vi "[ToBeTest] Complete Measurament RT.vi"() -> ()   [LabVIEW 2014]
uses:
  <vilib>/Platform/TimedLoop/XDataNode/timing_clust.ctl
  <vilib>/Platform/TimedLoop/XDataNode/nitl_modes.ctl
  <vilib>/Platform/TimedLoop/XDataNode/wakeup.ctl
  <vilib>/FPGAPlugInAG/sbRIO-9636/niLvFpga_Open_sbRIO-9636.vi
  <vilib>/rvi/interface/common/dynamic/niFpgaDynamicAddResources.vi
  <vilib>/FPGAPlugInAG/Dynamic/niLvFpga_Reset_Dynamic.vi
  <vilib>/Utility/error.llb/Error Cluster From Error Code.vi
  <vilib>/rvi/errors/niLvFpgaAdjustHostInterfaceError.vi
  <vilib>/rvi/interface/common/niFpgaWaitOnOcc.vi
  <vilib>/FPGAPlugInAG/Dynamic/niLvFpga_Run_Dynamic.vi
  <vilib>/FPGAPlugInAG/Dynamic/niLvFpga_Abort_Dynamic.vi
  <vilib>/FPGAPlugInAG/Dynamic/niLvFpga_Close_Dynamic.vi
  <vilib>/rvi/interface/nirviOpenFPGA/nirviOpenFPGA.xnode
  FPGA Bitfiles/LaserDistanceSen_FPGATarget_N-ParametricDoub_YVLbjAYtdP4.lvbitx
  FPGA Target/Test VIs/N-Parametric Double FFT Mesurament Test.vi
  <vilib>/rvi/interface/nirviMethod/nirviMethod.xnode
  <vilib>/rvi/interface/nirviReadWriteControl/nirviReadWriteControl.xnode
  <vilib>/platform/TimedLoop/XDataNode/XDataNode.xnode
  <vilib>/rvi/interface/nirviCloseFPGA/nirviCloseFPGA.xnode
  <vilib>/FPGAPlugInAG/Dynamic/niLvFpga_ConfigureFifo_Dynamic.vi
  <vilib>/rvi/errors/niLvFpgaMergeErrorWithErrorCode.vi
  <vilib>/FPGAPlugInAG/Dynamic/niLvFpga_StartFifo_Dynamic.vi
  <vilib>/rvi/interface/Simulation/niFpgaSimulationCallBeginRW.vi
  <vilib>/FPGAPlugInAG/Dynamic/niLvFpga_ReadFifo_Dynamic.vi
  <vilib>/Platform/TimedLoop/XDataNode/XDNodeRunTimeDep.lvlib
  NiFpgaLv.dll
  <vilib>/Analysis/NI_AALBase.lvlib
panel:
  in  "#movesignal":i32=10
  out "moving standard deviation rel":dbl format="%0.5f"
  out "moving mean":dbl format="%0.7f"
  out "StdDev Rel 1":dbl
  out "StdDev Rel 2":dbl
  out "Warning":bool
  out "Velocity (m/s)":dbl
  out "Distance (m)":dbl
  out "Mean Frequency":dbl
  out "Rise array size":i32
  out "Fall array size":i32
  out "Mean Frequency Rising (Hz)":dbl
  out "Mean Frequency Falling (Hz)":dbl
  in  "tieni premuto per":i32=1
  in  "Triangular Multiply Factor":dbl[](array[numeric])=[1.0, 0.8, 0.95, 0.85, 0.9]
  out "RISING Second Edge N-FFT":dbl[](graph)
  in  "Enable triangular scaling":bool=TRUE
  in  "Triangolo dritto?":bool
  out "FALLING First Edge N-FFT":dbl[](graph)
  in  "#Signals":u32(slide)=5 scale=1.0..5.0
  in  "stop":bool
  in  "Initial Latency points":u32(slide) scale=0.0..1249.0
  out "Elements Remaining FFT":u32
  out "Elements Remaining Signal":u32
  out "N-Signals":dbl[](graph)
  in  "Snapshot":bool
  in  "Windowing":T1(ring)
  in  "first bin":i32=5
  in  "last bin":i32=255
  in  "lower limit 2":u32(slide)=738 scale=625.0..738.0
  in  "lower limit 1":u32(slide)=113 scale=0.0..113.0
  # "OFFLINE parameters"
  # "Max Detection FFT bin range"
  # "WARNING:\nOnce pressed wait untill the end of operation"
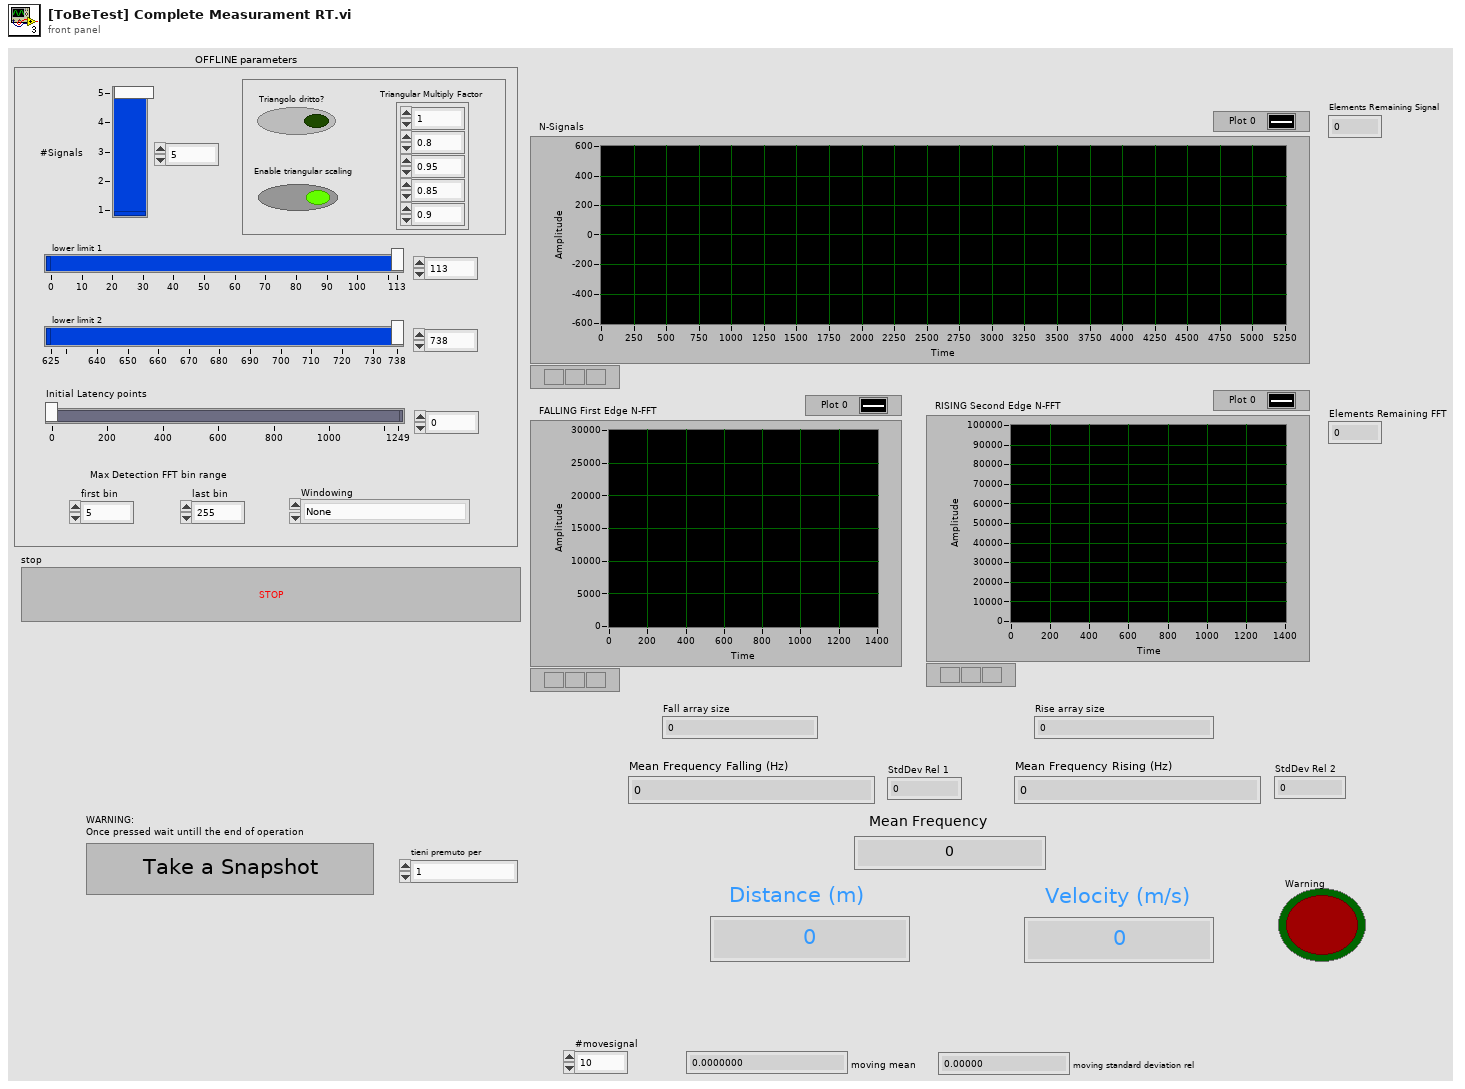
[diagram p1: front panel]
types:
  T1 = enum16{"None", "Hanning", "Hamming", "Blackman", "Blackman-Harris"}
  T2 = typedef "XDNodeRunTimeDep.lvlib/timing_clust.ctl" = cluster{"Expected End [f-1]":u64, "Actual End [f-1]":u64, "Finished Late? [f-1]":bool, "Expected End [i-1]":u64, "Actual End [i-1]":u64, "Finished Late? [i-1]":bool, "Expected Start [i]":u64, "Actual Start [i]":u64, "Expected Start [f]":u64, "Actual Start [f]":u64, "Source Name":string, "Structure Name":string, "Period":i64, "Deadline":i64, "Offset":i64, "Start":i64, "Priority":i32, "Timeout":i32, "Mode":T3, "Wakeup Reason":T4, "Error":errorcluster, "Source Type":string, "Secondary Source Type":string, "Global End Time":u64, "Global Start Time":u64, "Frame Duration":u64, "Iteration Duration":u64, "Assigned CPU":i32, "I/O Scan Engine Mode":u32}
  T3 = typedef "XDNodeRunTimeDep.lvlib/nitl_modes.ctl" = enum32{"No Change", "Process missed periods, maintain original phase", "Discard missed periods, maintain original phase", "Process missed periods, ignore original phase", "Discard missed periods, ignore original phase"}
  T4 = typedef "XDNodeRunTimeDep.lvlib/wakeup.ctl" = enum32{"Normal", "Aborted", "Asynchronous wakeup", "Timing source error", "Timed loop error", "Timeout"}
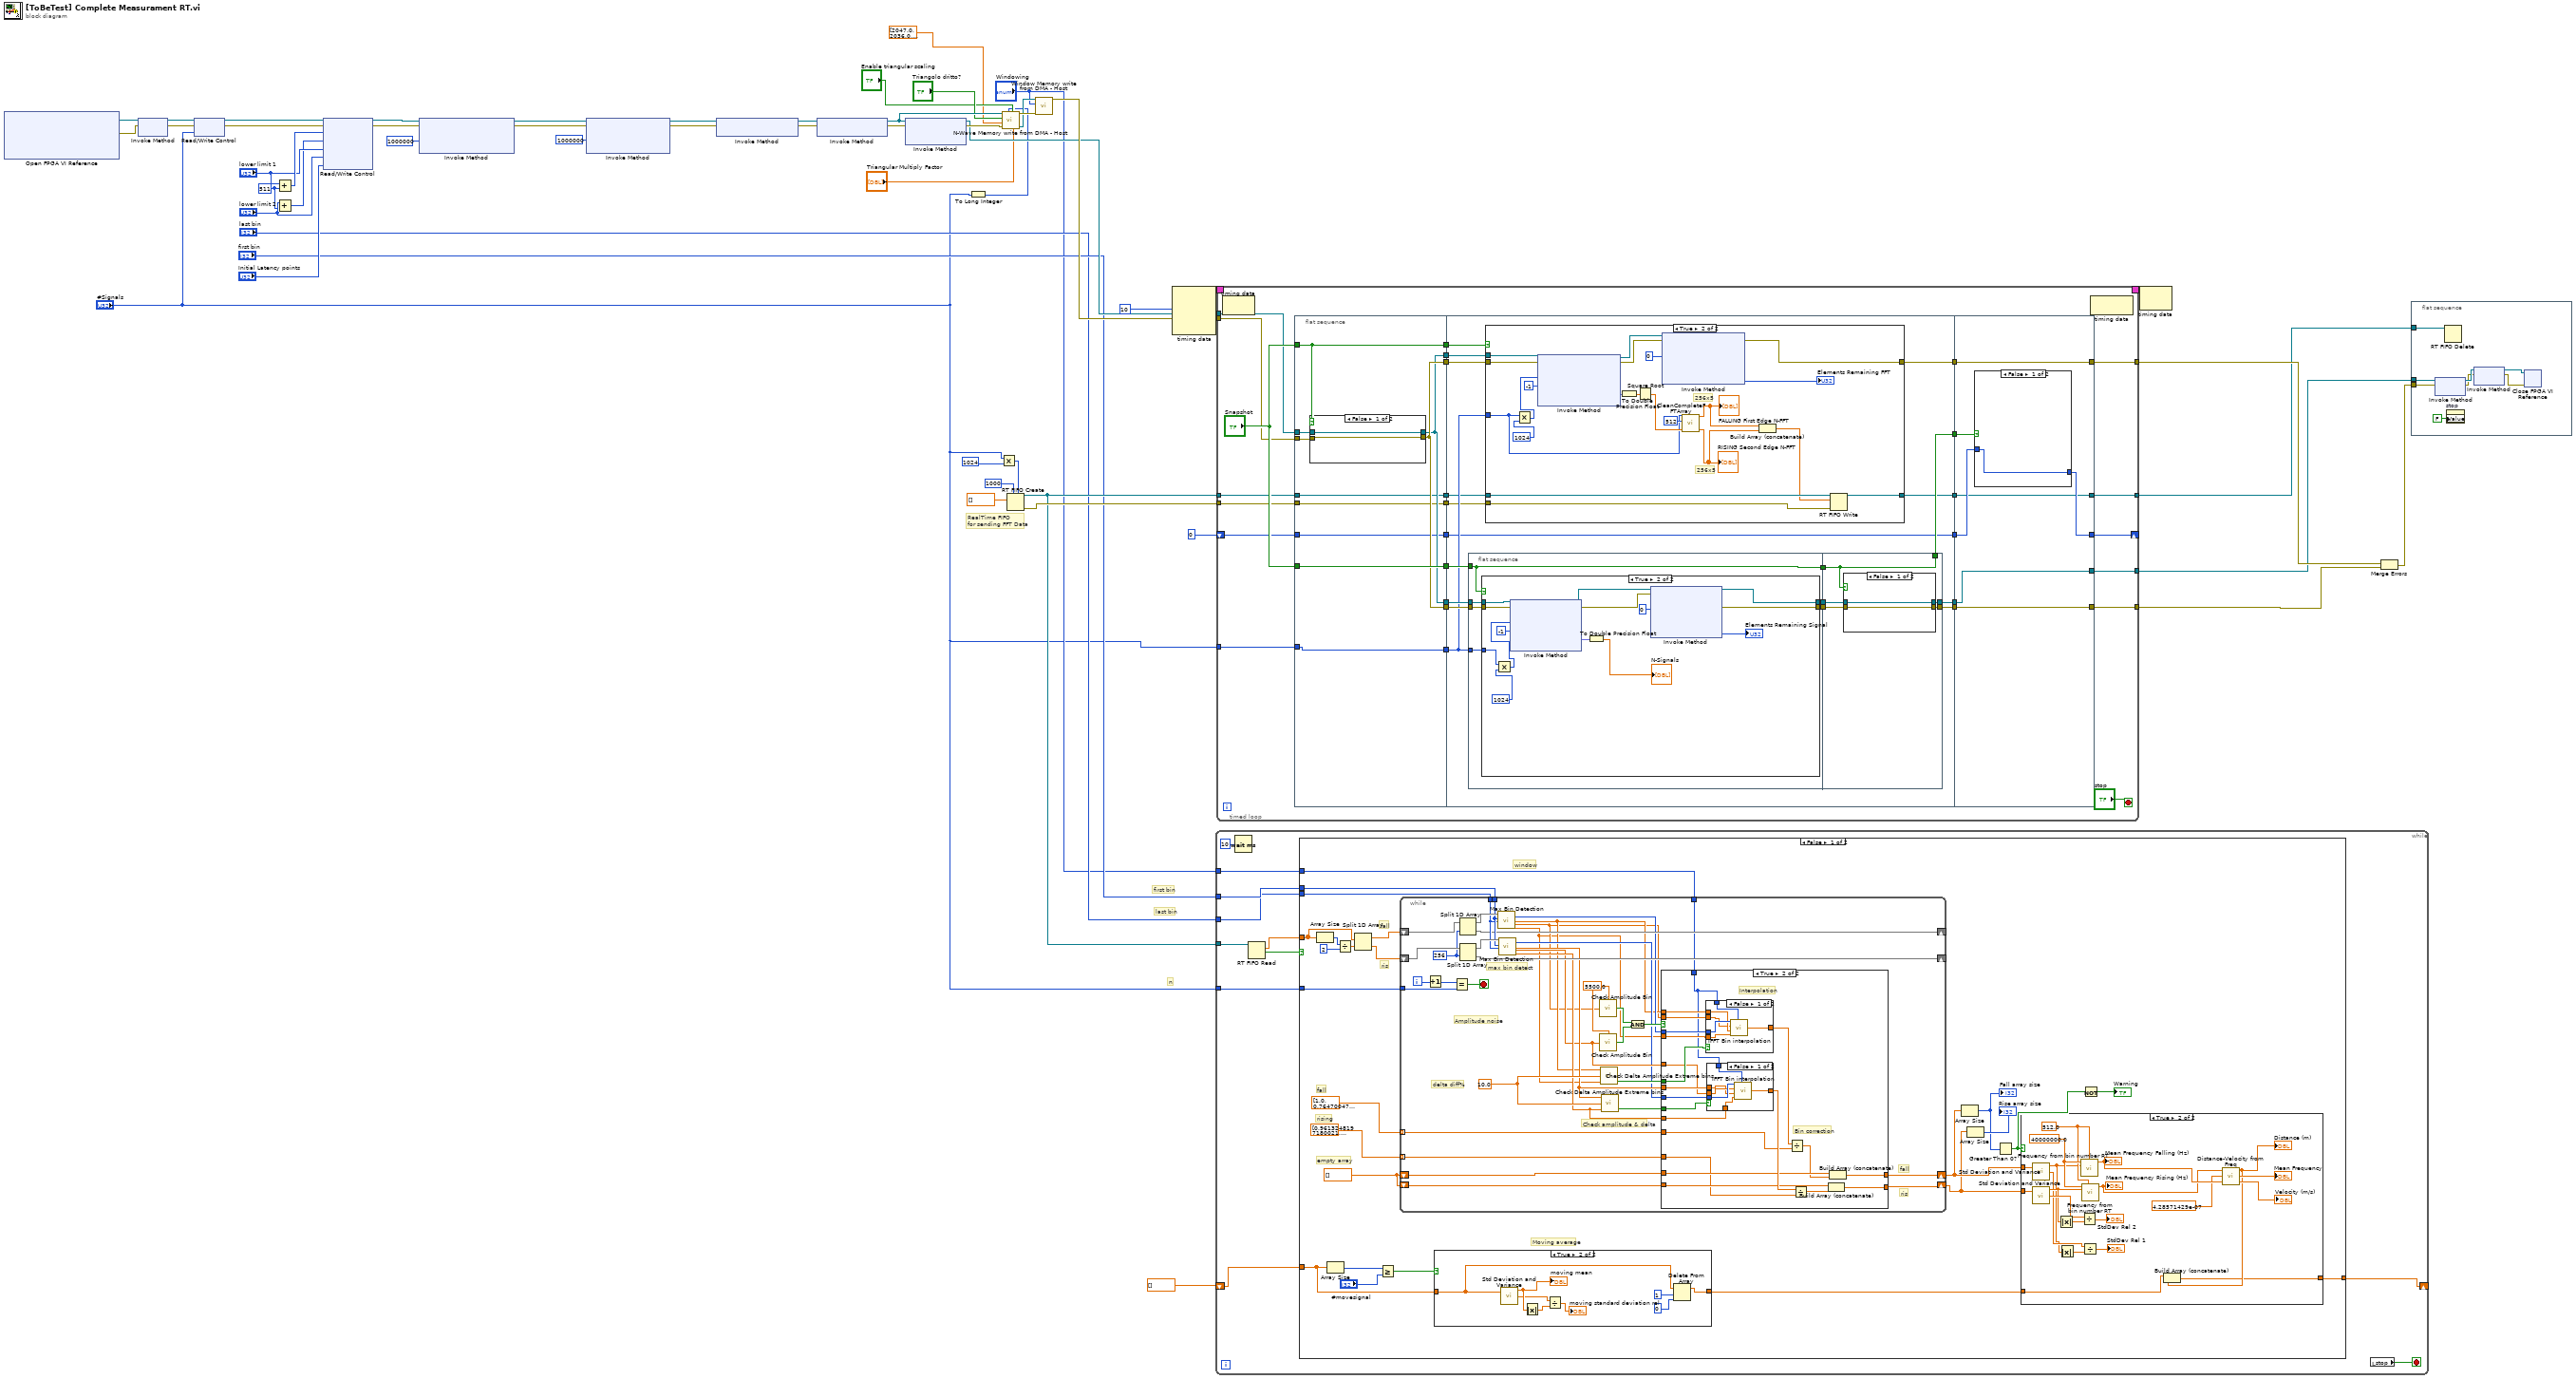
[diagram p0: block diagram]
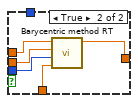
[diagram p5: hidden frame]
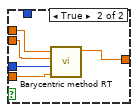
[diagram p6: hidden frame]
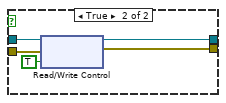
[diagram p8: hidden frame]
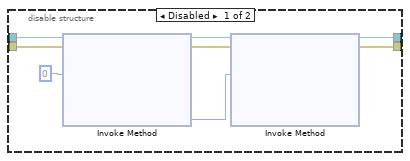
[diagram p10: hidden frame]
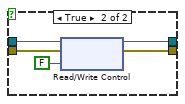
[diagram p11: hidden frame]
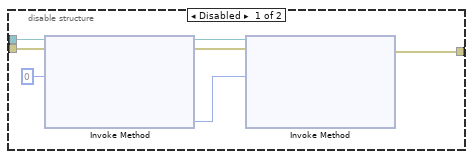
[diagram p13: hidden frame]
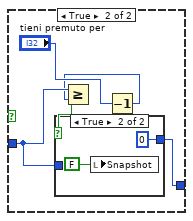
[diagram p14: hidden frame]
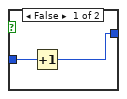
[diagram p15: hidden frame]
diagram:
  w50 = u32 511 ("y")
  # "n"
  # "last bin"
  # "first bin"
  # "RealTime FIFO \nfor sending FFT Data"
  n1 = xnode "Open FPGA VI Reference"() -> ("FPGA VI Reference Out"=w24:refnum<k20>, "error out"=w23:errorcluster)  [unwired: 2 in]
  n2 = xnode "Invoke Method"("FPGA VI Reference In"=w24, "error in"=w23) -> ("FPGA VI Reference Out"=w21:refnum<k20>, "error out"=w22:errorcluster)
  n3 = xnode "Read/Write Control"("FPGA VI Reference In"=w21, "error in"=w22, "n"="#Signals") -> ("FPGA VI Reference Out"=w20:refnum<k20>, "error out"=w19:errorcluster)
  n4 = Add(x="lower limit 1", y=w50) -> (x+y=w54:u32)
  n5 = Add(x="lower limit 2", y=w50) -> (x+y=w52:u32)
  n6 = xnode "Read/Write Control"("FPGA VI Reference In"=w20, "error in"=w19, "upper limit 1"=w54, "upper limit 2"=w52, "lower limit 1"="lower limit 1", "lower limit 2"="lower limit 2", "Latency points"="Initial Latency points") -> ("FPGA VI Reference Out"=w48:refnum<k20>, "error out"=w47:errorcluster)
  n7 = xnode "Invoke Method"("FPGA VI Reference In"=w48, "error in"=w47, "Requested Depth"=u32 1000000) -> ("FPGA VI Reference Out"=w35:refnum<k20>, "error out"=w36:errorcluster)  [unwired: 1 out]
  n8 = xnode "Invoke Method"("FPGA VI Reference In"=w35, "error in"=w36, "Requested Depth"=u32 1000000) -> ("FPGA VI Reference Out"=w42:refnum<k20>, "error out"=w43:errorcluster)  [unwired: 1 out]
  n9 = xnode "Invoke Method"("FPGA VI Reference In"=w42, "error in"=w43) -> ("FPGA VI Reference Out"=w33:refnum<k20>, "error out"=w34:errorcluster)
  n10 = xnode "Invoke Method"("FPGA VI Reference In"=w33, "error in"=w34) -> ("FPGA VI Reference Out"=w28:refnum<k20>, "error out"=w41:errorcluster)
  n11 = xnode "Invoke Method"("FPGA VI Reference In"=w28, "error in"=w41) -> ("FPGA VI Reference Out"=w29:refnum<k20>, "error out"=w32:errorcluster)  [unwired: 1 in]
  n12 = To Long Integer(number="#Signals") -> (32bit integer=w14:i32)
  n13 = Multiply(x="#Signals", y=u32 1024 ("elements in array (1)")) -> (x*y=w10:u32)
  n14 = call "N-Wave Memory write from DMA - Host.vi"("Triangular Multiply Factor"="Triangular Multiply Factor", "Enable triangular scaling"="Enable triangular scaling", "n"=w14, "error in"=w32, "Custom Triangular Signal (fal-ris)"=dbl[] [2047.0, 2036.0, 2024.0, 2013.0, 2002.0, 1990.0, 1979.0, 1968.0, 1956.0, 1945.0, 1934.0, 1923.0, 1912.0, 1900.0, 1889.0, 1878.0, 1867.0, 1856.0, 1845.0, 1833.0, 1822.0, 1811.0, 1800.0, 1789.0, 1778.0, 1767.0, 1756.0, 1745.0, 1734.0, 1723.0, 1712.0, 1702.0, 1691.0, 1680.0, 1669.0, 1658.0, 1647.0, 1636.0, 1626.0, 1615.0, 1604.0, 1593.0, 1583.0, 1572.0, 1561.0, 1550.0, 1540.0, 1529.0, 1518.0, 1508.0, 1497.0, 1487.0, 1476.0, 1465.0, 1455.0, 1444.0, 1434.0, 1423.0, 1413.0, 1402.0, 1392.0, 1381.0, 1371.0, 1360.0, 1350.0, 1340.0, 1329.0, 1319.0, 1309.0, 1298.0, 1288.0, 1278.0, 1267.0, 1257.0, 1247.0, 1237.0, 1226.0, 1216.0, 1206.0, 1196.0, 1186.0, 1176.0, 1165.0, 1155.0, 1145.0, 1135.0, 1125.0, 1115.0, 1105.0, 1095.0, 1085.0, 1075.0, 1065.0, 1055.0, 1045.0, 1035.0, 1025.0, 1015.0, 1006.0, 996.0, 986.0, 976.0, 966.0, 956.0, 947.0, 937.0, 927.0, 917.0, 908.0, 898.0, 888.0, 879.0, 869.0, 859.0, 850.0, 837.0, 826.0, 816.0, 804.0, 796.0, 788.0, 778.0, 769.0, 758.0, 750.0, 743.0, 733.0, 724.0, 717.0, 709.0, 701.0, 693.0, 686.0, 677.0, 669.0, 661.0, 653.0, 645.0, 638.0, 630.0, 622.0, 615.0, 607.0, 599.0, 592.0, 583.0, 576.0, 569.0, 561.0, 554.0, 547.0, 539.0, 532.0, 525.0, 518.0, 509.0, 501.0, 492.0, 486.0, 478.0, 471.0, 463.0, 456.0, 450.0, 442.0, 435.0, 429.0, 421.0, 415.0, 408.0, 401.0, 394.0, 388.0, 381.0, 375.0, 368.0, 361.0, 355.0, 349.0, 342.0, 336.0, 330.0, 323.0, 317.0, 311.0, 304.0, 298.0, 292.0, 286.0, 279.0, 273.0, 267.0, 261.0, 255.0, 249.0, 242.0, 236.0, 230.0, 224.0, 218.0, 212.0, 206.0, 200.0, 194.0, 187.0, 181.0, 175.0, 169.0, 163.0, 157.0, 150.0, 144.0, 138.0, 132.0, 125.0, 119.0, 113.0, 107.0, 101.0, 95.0, 88.0, 82.0, 77.0, 71.0, 65.0, 59.0, 53.0, 47.0, 41.0, 35.0, 29.0, 23.0, 18.0, 11.0, 6.0, 0.0, -6.0, -12.0, -18.0, -23.0, -29.0, -35.0, -41.0, -47.0, -52.0, -58.0, -64.0, -69.0, -75.0, -81.0, -87.0, -92.0, -98.0, -104.0, -109.0, -115.0, -121.0, -126.0, -132.0, -138.0, -144.0, -149.0, -155.0, -161.0, -166.0, -172.0, -177.0, -183.0, -189.0, -194.0, -200.0, -205.0, -211.0, -216.0, -222.0, -227.0, -233.0, -238.0, -244.0, -249.0, -255.0, -260.0, -266.0, -271.0, -277.0, -283.0, -288.0, -294.0, -299.0, -304.0, -310.0, -315.0, -321.0, -326.0, -331.0, -337.0, -342.0, -348.0, -353.0, -358.0, -364.0, -369.0, -375.0, -380.0, -385.0, -391.0, -396.0, -402.0, -407.0, -413.0, -418.0, -423.0, -429.0, -434.0, -439.0, -445.0, -450.0, -456.0, -461.0, -466.0, -472.0, -477.0, -483.0, -488.0, -493.0, -499.0, -504.0, -510.0, -515.0, -520.0, -526.0, -531.0, -537.0, -542.0, -548.0, -553.0, -558.0, -564.0, -569.0, -574.0, -580.0, -585.0, -590.0, -596.0, -601.0, -606.0, -612.0, -617.0, -622.0, -628.0, -633.0, -638.0, -644.0, -649.0, -654.0, -660.0, -665.0, -670.0, -676.0, -681.0, -686.0, -692.0, -697.0, -702.0, -708.0, -713.0, -718.0, -723.0, -729.0, -734.0, -739.0, -744.0, -750.0, -755.0, -760.0, -765.0, -771.0, -776.0, -781.0, -786.0, -792.0, -797.0, -802.0, -807.0, -812.0, -818.0, -823.0, -828.0, -833.0, -839.0, -844.0, -849.0, -854.0, -859.0, -865.0, -870.0, -875.0, -880.0, -885.0, -891.0, -896.0, -901.0, -906.0, -911.0, -916.0, -922.0, -927.0, -932.0, -937.0, -943.0, -948.0, -953.0, -958.0, -963.0, -969.0, -974.0, -979.0, -984.0, -989.0, -995.0, -1000.0, -1005.0, -1010.0, -1015.0, -1021.0, -1026.0, -1031.0, -1036.0, -1041.0, -1047.0, -1052.0, -1057.0, -1062.0, -1067.0, -1073.0, -1078.0, -1083.0, -1088.0, -1093.0, -1099.0, -1104.0, -1109.0, -1114.0, -1119.0, -1124.0, -1130.0, -1135.0, -1140.0, -1145.0, -1150.0, -1156.0, -1161.0, -1166.0, -1171.0, -1176.0, -1182.0, -1187.0, -1192.0, -1197.0, -1202.0, -1207.0, -1213.0, -1218.0, -1223.0, -1228.0, -1233.0, -1238.0, -1244.0, -1249.0, -1254.0, -1259.0, -1264.0, -1269.0, -1275.0, -1280.0, -1285.0, -1290.0, -1295.0, -1300.0, -1305.0, -1311.0, -1316.0, -1321.0, -1326.0, -1331.0, -1336.0, -1342.0, -1347.0, -1352.0, -1357.0, -1362.0, -1367.0, -1372.0, -1378.0, -1383.0, -1388.0, -1393.0, -1398.0, -1403.0, -1408.0, -1414.0, -1419.0, -1424.0, -1429.0, -1434.0, -1439.0, -1444.0, -1450.0, -1455.0, -1460.0, -1465.0, -1470.0, -1475.0, -1480.0, -1486.0, -1491.0, -1496.0, -1501.0, -1506.0, -1511.0, -1516.0, -1522.0, -1527.0, -1532.0, -1537.0, -1542.0, -1547.0, -1552.0, -1558.0, -1563.0, -1568.0, -1573.0, -1578.0, -1583.0, -1588.0, -1593.0, -1599.0, -1604.0, -1609.0, -1614.0, -1619.0, -1624.0, -1629.0, -1634.0, -1640.0, -1645.0, -1650.0, -1655.0, -1660.0, -1665.0, -1670.0, -1675.0, -1681.0, -1686.0, -1691.0, -1696.0, -1701.0, -1706.0, -1711.0, -1716.0, -1722.0, -1727.0, -1732.0, -1737.0, -1742.0, -1747.0, -1752.0, -1757.0, -1762.0, -1768.0, -1773.0, -1778.0, -1783.0, -1788.0, -1793.0, -1798.0, -1803.0, -1808.0, -1814.0, -1819.0, -1824.0, -1829.0, -1834.0, -1839.0, -1844.0, -1849.0, -1854.0, -1859.0, -1865.0, -1870.0, -1875.0, -1880.0, -1885.0, -1890.0, -1895.0, -1900.0, -1905.0, -1911.0, -1916.0, -1921.0, -1926.0, -1931.0, -1936.0, -1941.0, -1946.0, -1951.0, -1956.0, -1961.0, -1967.0, -1972.0, -1977.0, -1982.0, -1987.0, -1992.0, -1997.0, -2002.0, -2007.0, -2012.0, -2017.0, -2023.0, -2028.0, -2033.0, -2038.0, -2043.0, -2048.0, -2047.0, -2034.0, -2021.0, -2009.0, -1996.0, -1983.0, -1970.0, -1957.0, -1945.0, -1932.0, -1919.0, -1907.0, -1894.0, -1881.0, -1869.0, -1856.0, -1844.0, -1831.0, -1819.0, -1806.0, -1794.0, -1781.0, -1769.0, -1757.0, -1744.0, -1732.0, -1719.0, -1707.0, -1695.0, -1682.0, -1670.0, -1658.0, -1646.0, -1634.0, -1621.0, -1609.0, -1597.0, -1585.0, -1573.0, -1561.0, -1549.0, -1537.0, -1525.0, -1513.0, -1501.0, -1489.0, -1477.0, -1465.0, -1453.0, -1441.0, -1429.0, -1417.0, -1405.0, -1394.0, -1382.0, -1370.0, -1358.0, -1347.0, -1335.0, -1323.0, -1312.0, -1300.0, -1288.0, -1277.0, -1265.0, -1254.0, -1242.0, -1231.0, -1219.0, -1208.0, -1196.0, -1185.0, -1173.0, -1162.0, -1150.0, -1139.0, -1128.0, -1116.0, -1105.0, -1094.0, -1083.0, -1071.0, -1060.0, -1049.0, -1038.0, -1027.0, -1015.0, -1004.0, -993.0, -982.0, -971.0, -960.0, -949.0, -938.0, -927.0, -916.0, -905.0, -894.0, -883.0, -873.0, -862.0, -851.0, -840.0, -829.0, -819.0, -808.0, -797.0, -786.0, -776.0, -765.0, -754.0, -744.0, -733.0, -722.0, -712.0, -697.0, -685.0, -674.0, -661.0, -652.0, -643.0, -632.0, -622.0, -610.0, -602.0, -594.0, -583.0, -574.0, -566.0, -558.0, -550.0, -542.0, -534.0, -525.0, -516.0, -507.0, -499.0, -491.0, -483.0, -475.0, -467.0, -459.0, -451.0, -443.0, -435.0, -426.0, -419.0, -411.0, -404.0, -396.0, -388.0, -381.0, -373.0, -366.0, -359.0, -349.0, -341.0, -331.0, -325.0, -317.0, -309.0, -301.0, -295.0, -288.0, -280.0, -273.0, -266.0, -259.0, -252.0, -246.0, -239.0, -231.0, -225.0, -219.0, -212.0, -205.0, -199.0, -192.0, -186.0, -180.0, -173.0, -167.0, -161.0, -155.0, -148.0, -142.0, -136.0, -130.0, -124.0, -118.0, -112.0, -106.0, -100.0, -94.0, -88.0, -82.0, -76.0, -70.0, -64.0, -58.0, -52.0, -46.0, -40.0, -34.0, -28.0, -21.0, -15.0, -9.0, -3.0, 2.0, 9.0, 15.0, 21.0, 27.0, 33.0, 39.0, 45.0, 51.0, 57.0, 63.0, 69.0, 75.0, 81.0, 86.0, 92.0, 98.0, 103.0, 110.0, 116.0, 121.0, 127.0, 133.0, 138.0, 144.0, 149.0, 155.0, 161.0, 166.0, 172.0, 177.0, 183.0, 189.0, 194.0, 200.0, 205.0, 211.0, 216.0, 221.0, 227.0, 232.0, 238.0, 243.0, 249.0, 254.0, 259.0, 265.0, 270.0, 276.0, 281.0, 286.0, 292.0, 297.0, 303.0, 308.0, 314.0, 319.0, 324.0, 329.0, 335.0, 340.0, 345.0, 351.0, 356.0, 361.0, 366.0, 371.0, 377.0, 382.0, 387.0, 392.0, 397.0, 403.0, 408.0, 413.0, 418.0, 423.0, 429.0, 434.0, 439.0, 444.0, 449.0, 454.0, 459.0, 464.0, 469.0, 474.0, 479.0, 484.0, 489.0, 494.0, 499.0, 504.0, 509.0, 514.0, 520.0, 525.0, 530.0, 535.0, 540.0, 545.0, 550.0, 555.0, 560.0, 565.0, 570.0, 575.0, 580.0, 585.0, 590.0, 595.0, 600.0, 605.0, 610.0, 615.0, 620.0, 625.0, 630.0, 636.0, 641.0, 646.0, 651.0, 656.0, 661.0, 666.0, 671.0, 676.0, 681.0, 686.0, 691.0, 696.0, 701.0, 706.0, 711.0, 716.0, 721.0, 726.0, 731.0, 736.0, 741.0, 746.0, 751.0, 756.0, 761.0, 765.0, 770.0, 775.0, 780.0, 785.0, 790.0, 795.0, 800.0, 805.0, 810.0, 815.0, 820.0, 825.0, 829.0, 834.0, 839.0, 844.0, 849.0, 854.0, 859.0, 864.0, 868.0, 873.0, 878.0, 883.0, 888.0, 893.0, 897.0, 902.0, 907.0, 912.0, 917.0, 921.0, 926.0, 931.0, 936.0, 941.0, 945.0, 950.0, 955.0, 960.0, 965.0, 969.0, 974.0, 979.0, 984.0, 988.0, 993.0, 998.0, 1003.0, 1007.0, 1012.0, 1017.0, 1022.0, 1027.0, 1031.0, 1036.0, 1041.0, 1046.0, 1051.0, 1055.0, 1060.0, 1065.0, 1070.0, 1075.0, 1079.0, 1084.0, 1089.0, 1094.0, 1098.0, 1103.0, 1108.0, 1113.0, 1118.0, 1122.0, 1127.0, 1132.0, 1137.0, 1141.0, 1146.0, 1151.0, 1156.0, 1161.0, 1165.0, 1170.0, 1175.0, 1180.0, 1184.0, 1189.0, 1194.0, 1199.0, 1204.0, 1208.0, 1213.0, 1218.0, 1223.0, 1227.0, 1232.0, 1237.0, 1242.0, 1246.0, 1251.0, 1256.0, 1261.0, 1265.0, 1270.0, 1275.0, 1280.0, 1284.0, 1289.0, 1294.0, 1299.0, 1303.0, 1308.0, 1313.0, 1318.0, 1322.0, 1327.0, 1332.0, 1336.0, 1341.0, 1346.0, 1351.0, 1355.0, 1360.0, 1365.0, 1370.0, 1374.0, 1379.0, 1384.0, 1388.0, 1393.0, 1398.0, 1403.0, 1407.0, 1412.0, 1417.0, 1421.0, 1426.0, 1431.0, 1436.0, 1440.0, 1445.0, 1450.0, 1454.0, 1459.0, 1464.0, 1469.0, 1473.0, 1478.0, 1483.0, 1487.0, 1492.0, 1497.0, 1502.0, 1506.0, 1511.0, 1516.0, 1520.0, 1525.0, 1530.0, 1535.0, 1539.0, 1544.0, 1549.0, 1553.0, 1558.0, 1563.0, 1567.0, 1572.0, 1577.0, 1582.0, 1586.0, 1591.0, 1596.0, 1600.0, 1605.0, 1610.0, 1614.0, 1619.0, 1624.0, 1628.0, 1633.0, 1638.0, 1643.0, 1647.0, 1652.0, 1657.0, 1661.0, 1666.0, 1671.0, 1675.0, 1680.0, 1685.0, 1689.0, 1694.0, 1699.0, 1703.0, 1708.0, 1713.0, 1717.0, 1722.0, 1727.0, 1731.0, 1736.0, 1741.0, 1746.0, 1750.0, 1755.0, 1760.0, 1764.0, 1769.0, 1774.0, 1778.0, 1783.0, 1788.0, 1792.0, 1797.0, 1802.0, 1806.0, 1811.0, 1816.0, 1820.0, 1825.0, 1830.0, 1834.0, 1839.0, 1844.0, 1848.0, 1853.0, 1858.0, 1862.0, 1867.0, 1871.0, 1876.0, 1881.0, 1885.0, 1890.0, 1895.0, 1899.0, 1904.0, 1909.0, 1913.0, 1918.0, 1923.0, 1927.0, 1932.0, 1937.0, 1941.0, 1946.0, 1951.0, 1955.0, 1960.0, 1965.0, 1969.0, 1974.0, 1978.0, 1983.0, 1988.0, 1992.0, 1997.0, 2002.0, 2006.0, 2011.0, 2016.0, 2020.0, 2025.0, 2029.0, 2034.0, 2039.0, 2043.0, 2048.0] ("Complete SkewTri"), "Triangolo dritto?"="Triangolo dritto?", "FPGA VI Reference In"=w28) -> ("FPGA VI Reference Out"=w30:refnum<k20>, "error out"=w31:errorcluster)  [unwired: 2 in, 1 out]
  n15 = RT FIFO Create(1:dbl[] [] ("double precision float"), 4:u32 1000 ("size (10)"), 6:w10) -> (8:w7:refnum<k33>, 11:w8:errorcluster)  [unwired: 5 in, 1 out]
  n16 = call "Window Memory write from DMA - Host.vi"("error in"=w31, "Enum"="Windowing", "FPGA VI Reference In"=w30) -> ("error out"=w49:errorcluster)  [unwired: 5 in, 3 out]
  n17 = node-c288(i64 10 ("Period")) -> (w27:T2)  [unwired: 3 in]
  n18 = while {
    tunnel: w7 -> [w64]
    tunnel: "first bin" -> [w61]
    tunnel: "last bin" -> [w60]
    tunnel: "Windowing" -> [w59]
    tunnel: "#Signals" -> [w58]
    shift-right: [w55] -> _
    shift-left: dbl[] [] ("appended array") -> [w56]
    stop <- w57 stop-if-true
    n19 = Wait (ms)(milliseconds to wait=u32 10 ("millisecond multiple")) -> ()  [unwired: 1 out]
    n20 = RT FIFO Read(0:w64) -> (9:w62:dbl[], 10:w63:bool)  [unwired: 3 in, 3 out]
    n21 = case shown="False" w63 {
      tunnel: w62 -> [w90 _]
      tunnel: w61 -> [w86 _]
      tunnel: w60 -> [w85 _]
      tunnel: w59 -> [w84 _]
      tunnel: w58 -> [w81 _]
      tunnel: w56 -> [w70 w201]
      tunnel: [w68 w201] -> w55
      frame False {
        w80 = dbl[] [] ("appended array")
        # "rising"
        # "fall"
        # "Moving average"
        # "empty array"
        # "window"
        # "ris"
        # "fall"
        n22 = Array Size(array=w90) -> (size(s)=w88:i32)
        n23 = Array Size(array=w70) -> (size(s)=w73:i32)
        n24 = Divide(x=w88, y=2) -> (x/y=w89:dbl)
        n25 = Split 1D Array(array=w90, index=w89) -> (first subarray=w82:dbl[], second subarray=w83:dbl[])
        n26 = Greater Or Equal?(x=w73, y="#movesignal") -> (x >= y?=w72:bool)
        n27 = while {
          shift-right: [w143] -> _
          shift-left: w82 -> [w155]
          shift-right: [w144] -> _
          shift-left: w83 -> [w154]
          tunnel: w86 -> [w151]
          tunnel: w85 -> [w150]
          tunnel: w84 -> [w127]
          tunnel: w81 -> [w148]
          shift-right: [w126] -> w79
          shift-left: w80 -> [w124]
          shift-right: [w125] -> w78
          shift-left: w80 -> [w123]
          tunnel: dbl[] [1.0, 0.7647004729921506, 0.9587386483466616, 0.823312577391412, 0.8946731320619146] ("mean factor 1") -> [w122] mode=indexing
          tunnel: dbl[] [0.9613248197180021, 0.8004726992011919, 0.9202842728499455, 0.8411537208279052, 0.8795877616861416] ("mean factor 2") -> [w121] mode=indexing
          i -> [w145]
          stop <- w149 stop-if-true
          w141 = 10.0 ("Max Difference %")
          w142 = 5500.0 ("Threshold Amp")
          w147 = 256 ("x")
          # "delta diff%"
          # "ris"
          # "fall"
          # "max bin detect"
          # "Check amplitude & delta"
          # "Amplitude noise"
          n28 = Increment(x=w145) -> (x+1=w146:i32)
          n29 = Equal?(x=w146, y=w148) -> (x = y?=w149:bool)
          n30 = Split 1D Array(array=w155, index=w147) -> (first subarray=w153:dbl[], second subarray=w143:dbl[])
          n31 = Split 1D Array(array=w154, index=w147) -> (first subarray=w152:dbl[], second subarray=w144:dbl[])
          n32 = call "Max Bin Detection.vi"("FFT Array"=w153, "Init Discard Bins"=w151, "Last Discard Bins"=w150) -> ("Max Bin"=w131:i32, "Prev Max Amp"=w130:dbl, "Max Amp"=w129:dbl, "Succ Max Amp"=w128:dbl)  [unwired: 11 in, 2 out]
          n33 = call "Max Bin Detection.vi"("FFT Array"=w152, "Init Discard Bins"=w151, "Last Discard Bins"=w150) -> ("Max Bin"=w132:i32, "Prev Max Amp"=w135:dbl, "Max Amp"=w133:dbl, "Succ Max Amp"=w134:dbl)  [unwired: 11 in, 2 out]
          n34 = call "Check Amplitude Bin.vi"("Threshold Amp"=w142, "Max Amp"=w129) -> ("Check Amp Ok?"=w140:bool)  [unwired: 2 in]
          n35 = call "Check Amplitude Bin.vi"("Threshold Amp"=w142, "Max Amp"=w133) -> ("Check Amp Ok?"=w139:bool)  [unwired: 2 in]
          n36 = call "Check Delta Amplitude Extreme bins.vi"("Succ Max Amp"=w128, "Max Difference %"=w141, "Prev Max Amp"=w130) -> ("Check Delta Amp Ok?"=w137:bool)  [unwired: 1 in, 1 out]
          n37 = call "Check Delta Amplitude Extreme bins.vi"("Succ Max Amp"=w134, "Max Difference %"=w141, "Prev Max Amp"=w135) -> ("Check Delta Amp Ok?"=w136:bool)  [unwired: 1 in, 1 out]
          n38 = And(x=w140, y=w139) -> (x .and. y?=w138:bool)
          n39 = case shown="True" w138 {
            tunnel: w137 -> [_ w178]
            tunnel: w136 -> [_ w177]
            tunnel: w135 -> [_ w176]
            tunnel: w134 -> [_ w175]
            tunnel: w133 -> [_ w174]
            tunnel: w132 -> [_ w173]
            tunnel: w131 -> [_ w172]
            tunnel: w130 -> [_ w171]
            tunnel: w129 -> [_ w170]
            tunnel: w128 -> [_ w169]
            tunnel: w127 -> [_ w168]
            tunnel: [w157 w165] -> w126
            tunnel: [w156 w164] -> w125
            tunnel: w124 -> [w157 w163]
            tunnel: w123 -> [w156 w162]
            tunnel: w122 -> [_ w160]
            tunnel: w121 -> [_ w158]
            frame False {
            }
            frame True {
              # "Bin correction"
              # "Interpolation"
              n40 = case shown="False" w178 {
                tunnel: w172 -> [w194 w200]
                tunnel: w171 -> [w192 w199]
                tunnel: w170 -> [w191 w198]
                tunnel: w169 -> [w190 w197]
                tunnel: [w193 w196] -> w167
                tunnel: w168 -> [w195 _]
                frame False {
                  n41 = call "IFFT Bin interpolation.vi"("Max Bin"=w194, "Max Amp"=w191, "Prev Max Amp"=w192, "Succ Max Amp"=w190, "Windowing"=w195) -> ("Interpolate Bin"=w193:dbl)
                }
                frame True {
                  n42 = call "Barycentric method RT.vi"("Next Amp"=w197, "Max Bin"=w200, "Max Amp"=w198, "Prev Amp"=w199) -> ("Bin"=w196:dbl)  [unwired: 7 in]
                }
              }
              n43 = case shown="False" w177 {
                tunnel: w176 -> [w180 w189]
                tunnel: w175 -> [w179 w188]
                tunnel: w174 -> [w181 w187]
                tunnel: w173 -> [w183 w186]
                tunnel: [w182 w185] -> w166
                tunnel: w168 -> [w184 _]
                frame False {
                  n44 = call "IFFT Bin interpolation.vi"("Max Bin"=w183, "Max Amp"=w181, "Prev Max Amp"=w180, "Succ Max Amp"=w179, "Windowing"=w184) -> ("Interpolate Bin"=w182:dbl)
                }
                frame True {
                  n45 = call "Barycentric method RT.vi"("Next Amp"=w188, "Max Bin"=w186, "Max Amp"=w187, "Prev Amp"=w189) -> ("Bin"=w185:dbl)  [unwired: 7 in]
                }
              }
              n46 = Divide(x=w167, y=w160) -> (x/y=w161:dbl)
              n47 = Divide(x=w166, y=w158) -> (x/y=w159:dbl)
              n48 = Build Array (concatenate)(w162, w159) -> (w164:dbl[])
              n49 = Build Array (concatenate)(w163, w161) -> (w165:dbl[])
            }
          }
        }
        n50 = case shown="True" w72 {
          tunnel: w70 -> [w91 w95]
          tunnel: [w91 w92] -> w69
          frame False {
          }
          frame True {
            n51 = call <vilib>:"Std Deviation and Variance.vi"("X"=w95) -> ("mean"=w99:dbl, "standard deviation"=w97:dbl)  [unwired: 1 in, 1 out]
            "moving mean" <- w99
            n52 = Absolute Value(x=w99) -> (abs(x)=w98:dbl)
            n53 = Divide(x=w97, y=w98) -> (x/y=→"moving standard deviation rel":dbl)
            n54 = Delete From Array(array=w95, length=1, index=0) -> (array with subset deleted=w92:dbl[])  [unwired: 1 out]
          }
        }
        n55 = Array Size(array=w79) -> (size(s)=w76:i32)
        "Fall array size" <- w76
        n56 = Array Size(array=w78) -> (size(s)=→"Rise array size":i32)
        n57 = Greater Than 0?(x=w76) -> (x > 0?=w74:bool)
        n58 = case shown="True" w74 {
          tunnel: w79 -> [_ w118]
          tunnel: w78 -> [_ w117]
          tunnel: w69 -> [w100 w103]
          tunnel: [w100 w101] -> w68
          frame False {
          }
          frame True {
            w119 = 512.0 ("FFT size")
            w120 = 40000000.0 ("Sample Rate (S/s)")
            n59 = call <vilib>:"Std Deviation and Variance.vi"("X"=w118) -> ("mean"=w104:dbl, "standard deviation"=w105:dbl)  [unwired: 1 in, 1 out]
            n60 = call <vilib>:"Std Deviation and Variance.vi"("X"=w117) -> ("mean"=w109:dbl, "standard deviation"=w111:dbl)  [unwired: 1 in, 1 out]
            n61 = Absolute Value(x=w109) -> (abs(x)=w110:dbl)
            n62 = Absolute Value(x=w104) -> (abs(x)=w106:dbl)
            n63 = call "Frequency from bin number RT.vi"("FFT size"=w119, "Bin number"=w104, "Sample Rate (S/s)"=w120) -> ("Detected Frequency (Hz)"=w116:dbl)  [unwired: 8 in]
            "Mean Frequency Falling (Hz)" <- w116
            n64 = Divide(x=w111, y=w110) -> (x/y=→"StdDev Rel 2":dbl)
            n65 = call "Frequency from bin number RT.vi"("FFT size"=w119, "Bin number"=w109, "Sample Rate (S/s)"=w120) -> ("Detected Frequency (Hz)"=w115:dbl)  [unwired: 8 in]
            "Mean Frequency Rising (Hz)" <- w115
            n66 = Divide(x=w105, y=w106) -> (x/y=→"StdDev Rel 1":dbl)
            n67 = call "Distance-Velocity from Freq.vi"("freq_rising"=w115, "Empirical Distance Costant"=4.28571429e-07, "freq_falling"=w116) -> ("Distance (m)"=w102:dbl, "Mean Frequency"=→"Mean Frequency":dbl, "Velocity (m/s)"=→"Velocity (m/s)":dbl)  [unwired: 2 in]
            "Distance (m)" <- w102
            n68 = Build Array (concatenate)(w103, w102) -> (w101:dbl[])
          }
        }
        n69 = Not(x=w74) -> (.not. x?=→"Warning":bool)
      }
      frame True {
      }
    }
    n70 = local read "stop"() -> (w57:bool)
  }
  n71 = timed-loop {
    tunnel: w29 -> [w226]
    tunnel: w49 -> [w227]
    tunnel: [w229] -> w40
    tunnel: [w230] -> w39
    tunnel: [w215] -> w37
    tunnel: "#Signals" -> [w212]
    timing: w27 -> [_]
    timing-out: [_] -> w26
    shift-right: [w208] -> _
    shift-left: 0 -> [w211]
    tunnel: w7 -> [w207]
    tunnel: w8 -> [w204]
    tunnel: [w202] -> w2
    stop <- "stop" stop-if-true
    n72 = node-c288() -> ()  [unwired: 1 in, 1 out]
    n73 = flat-sequence {
      tunnel: w226 -> [w239]
      tunnel: w227 -> [w240]
      tunnel: "Snapshot" -> [w237]
      tunnel: "Snapshot" -> [w242]
      tunnel: [w241] -> w225
      tunnel: [w242] -> w224
      tunnel: [w237] -> w223
      tunnel: [w241] -> w222
      tunnel: [w238] -> w221
      tunnel: [w238] -> w220
      tunnel: [w236] -> w213
      tunnel: w212 -> [w236]
      tunnel: w211 -> [w235]
      tunnel: [w235] -> w210
      tunnel: w207 -> [w234]
      tunnel: [w234] -> w206
      tunnel: [w233] -> w205
      tunnel: w204 -> [w233]
      tunnel: w225 -> [w263]
      tunnel: w224 -> [w257]
      tunnel: w223 -> [w260]
      tunnel: w222 -> [w259]
      tunnel: w221 -> [w258]
      tunnel: w220 -> [w264]
      tunnel: [w262] -> w219
      tunnel: [w261] -> w218
      tunnel: [w256] -> w217
      tunnel: [w255] -> w214
      tunnel: w213 -> [w254]
      tunnel: w210 -> [w253]
      tunnel: [w253] -> w209
      tunnel: w206 -> [w252]
      tunnel: w205 -> [w251]
      tunnel: [w250] -> w203
      tunnel: [w352] -> w229
      tunnel: [w353] -> w230
      tunnel: w219 -> [w353]
      tunnel: w218 -> [w352]
      tunnel: w217 -> [w350]
      tunnel: [w351] -> w215
      tunnel: w214 -> [w351]
      tunnel: w209 -> [w349]
      tunnel: [w348] -> w208
      tunnel: w203 -> [w347]
      tunnel: [w347] -> w202
      frame #0 {
        n74 = case shown="False" w237 {
          tunnel: [w243 w249] -> w241
          tunnel: w240 -> [w243 w248]
          tunnel: w239 -> [w244 w247]
          tunnel: [w244 w246] -> w238
          frame False {
          }
          frame True {
            n75 = xnode "Read/Write Control"("FPGA VI Reference In"=w247, "error in"=w248, "snapshot"=TRUE) -> ("FPGA VI Reference Out"=w246:refnum<k20>, "error out"=w249:errorcluster)
          }
        }
      }
      frame #1 {
        n76 = flat-sequence {
          tunnel: w264 -> [w273]
          tunnel: w263 -> [w272]
          tunnel: w257 -> [w269]
          tunnel: [w271] -> w267
          tunnel: [w270] -> w266
          tunnel: [w269] -> w265
          tunnel: w254 -> [w268]
          tunnel: [w304] -> w261
          tunnel: w267 -> [w306]
          tunnel: w266 -> [w305]
          tunnel: w265 -> [w303]
          tunnel: [w303] -> w256
          tunnel: [w302] -> w255
          frame #0 {
            n77 = case shown="True" w269 {
              tunnel: w273 -> [w277 w301]
              tunnel: w272 -> [w276 w300]
              tunnel: [w275 w299] -> w270
              tunnel: [w274 w298] -> w271
              tunnel: w268 -> [_ w297]
              frame False {
                n78 = disable-structure shown="Enabled" {
                  disable-tunnel: w277 -> [w284 w287]
                  disable-tunnel: w276 -> [w282 w286]
                  disable-tunnel: [w281 w286] -> w275
                  disable-tunnel: [w278 w287] -> w274
                  frame Disabled {
                    n79 = xnode "Invoke Method"("FPGA VI Reference In"=w284, "error in"=w282, "Number of Elements"=u32 0) -> ("FPGA VI Reference Out"=w280:refnum<k20>, "error out"=w279:errorcluster, "Elements Remaining"=w283:u32)  [unwired: 1 in, 1 out]
                    n80 = xnode "Invoke Method"("FPGA VI Reference In"=w280, "error in"=w279, "Number of Elements"=w283) -> ("FPGA VI Reference Out"=w278:refnum<k20>, "error out"=w281:errorcluster)  [unwired: 1 in, 2 out]
                  }
                  frame Enabled {
                  }
                }
              }
              frame True {
                n81 = Multiply(x=w297, y=u32 1024 ("Number of Elements")) -> (x*y=w291:u32)
                n82 = xnode "Invoke Method"("FPGA VI Reference In"=w301, "error in"=w300, "Number of Elements"=w291, "Timeout (ms)"=-1) -> ("FPGA VI Reference Out"=w294:refnum<k20>, "error out"=w293:errorcluster, "Data"=w296:fxp<+/-,12,12>[])  [unwired: 1 out]
                n83 = To Double Precision Float(number=w296) -> (double precision float=→"N-Signals":dbl[])
                n84 = xnode "Invoke Method"("FPGA VI Reference In"=w294, "error in"=w293, "Number of Elements"=u32 0) -> ("FPGA VI Reference Out"=w298:refnum<k20>, "error out"=w299:errorcluster, "Elements Remaining"=→"Elements Remaining Signal":u32)  [unwired: 1 in, 1 out]
              }
            }
          }
          frame #1 {
            n85 = case shown="False" w303 {
              tunnel: [w308 w311] -> w304
              tunnel: w306 -> [w307 w312]
              tunnel: w305 -> [w308 w310]
              tunnel: [w307 w309] -> w302
              frame False {
              }
              frame True {
                n86 = xnode "Read/Write Control"("FPGA VI Reference In"=w312, "error in"=w310, "snapshot"=FALSE) -> ("FPGA VI Reference Out"=w309:refnum<k20>, "error out"=w311:errorcluster)
              }
            }
          }
        }
        n87 = case shown="True" w260 {
          tunnel: w258 -> [w317 w345]
          tunnel: w259 -> [w316 w346]
          tunnel: [w315 w344] -> w262
          tunnel: w254 -> [_ w332]
          tunnel: w252 -> [w314 w330]
          tunnel: w251 -> [_ w329]
          tunnel: [w314 w327] -> w250
          frame False {
            n88 = disable-structure shown="Enabled" {
              disable-tunnel: w317 -> [w323 _]
              disable-tunnel: w316 -> [w320 w325]
              disable-tunnel: [w319 w325] -> w315
              frame Disabled {
                n89 = xnode "Invoke Method"("FPGA VI Reference In"=w323, "error in"=w320, "Number of Elements"=u32 0) -> ("FPGA VI Reference Out"=w321:refnum<k20>, "error out"=w318:errorcluster, "Elements Remaining"=w322:u32)  [unwired: 1 in, 1 out]
                n90 = xnode "Invoke Method"("FPGA VI Reference In"=w321, "error in"=w318, "Number of Elements"=w322) -> ("error out"=w319:errorcluster)  [unwired: 1 in, 3 out]
              }
              frame Enabled {
              }
            }
          }
          frame True {
            # "256x5"
            # "256x5"
            n91 = Multiply(x=w332, y=u32 1024 ("Number of Elements")) -> (x*y=w336:u32)
            n92 = xnode "Invoke Method"("FPGA VI Reference In"=w345, "error in"=w346, "Number of Elements"=w336, "Timeout (ms)"=-1) -> ("FPGA VI Reference Out"=w340:refnum<k20>, "error out"=w341:errorcluster, "Data"=w343:fxp<+,44,44>[])  [unwired: 1 out]
            n93 = To Double Precision Float(number=w343) -> (double precision float=w342:dbl[])
            n94 = Square Root(x=w342) -> (sqrt(x)=w333:dbl[])
            n95 = xnode "Invoke Method"("FPGA VI Reference In"=w340, "error in"=w341, "Number of Elements"=u32 0) -> ("error out"=w344:errorcluster, "Elements Remaining"=→"Elements Remaining FFT":u32)  [unwired: 1 in, 2 out]
            n96 = call "CleanCompleteFFTArray.vi"("Complete FFT Array"=w333, "FFT Size"=512, "#Signals"=w332) -> ("Second Edge Array"=w331:dbl[], "First Edge Array"=w326:dbl[])  [unwired: 7 in]
            "FALLING First Edge N-FFT" <- w326
            "RISING Second Edge N-FFT" <- w331
            n97 = Build Array (concatenate)(w326, w331) -> (w328:dbl[])
            n98 = RT FIFO Write(0:w330, 1:w328, 3:w329) -> (8:w327:refnum<k33>)  [unwired: 2 in, 3 out]
          }
        }
      }
      frame #2 {
        n99 = case shown="False" w350 {
          tunnel: w349 -> [w354 w358]
          tunnel: [w354 w359] -> w348
          frame False {
          }
          frame True {
            n100 = Decrement(x="tieni premuto per") -> (x-1=w355:i32)
            n101 = Greater Or Equal?(x=w358, y=w355) -> (x >= y?=w357:bool)
            n102 = case shown="True" w357 {
              tunnel: w358 -> [w360 _]
              tunnel: [w361 0] -> w359
              frame False {
                n103 = Increment(x=w360) -> (x+1=w361:i32)
              }
              frame True {
                n104 = local write "Snapshot"(FALSE ("Snapshot")) -> ()
              }
            }
          }
        }
      }
    }
    n105 = node-c288() -> ()  [unwired: 1 in, 1 out]
  }
  n106 = node-c288(w26) -> ()  [unwired: 1 out]
  n107 = Merge Errors(w39, w40) -> (w44:errorcluster)
  n108 = flat-sequence {
    tunnel: w44 -> [w371]
    tunnel: w37 -> [w366]
    tunnel: w2 -> [w364]
    frame #0 {
      n109 = xnode "Invoke Method"("FPGA VI Reference In"=w366, "error in"=w371) -> ("FPGA VI Reference Out"=w368:refnum<k20>, "error out"=w367:errorcluster)
      n110 = RT FIFO Delete(0:w364) -> ()  [unwired: 2 in, 1 out]
      n111 = property on="stop" class="Bool (strict)"("Value"=FALSE ("stop")) -> ()  [unwired: 2 in, 2 out]
      n112 = xnode "Invoke Method"("FPGA VI Reference In"=w368, "error in"=w367) -> ("FPGA VI Reference Out"=w369:refnum<k20>, "error out"=w370:errorcluster)
      n113 = xnode "Close FPGA VI Reference"("FPGA VI Reference In"=w369, "error in"=w370) -> ()  [unwired: 1 out]
    }
  }
